vi "CR-SaveImage -CCD3NG.vi"(6 "CCD Name":string(combo), 8 "error in (no error)":errorcluster, 9 "Image in":T1(plugin-control), 10 "布尔":bool=TRUE, 11 "基路径":path) -> (0 "error out":errorcluster)   [LabVIEW 2017]
panel:
  out "连接的字符串":string
  # "D:\\Data\\History Image\\20190228\\CCD3\\Image"
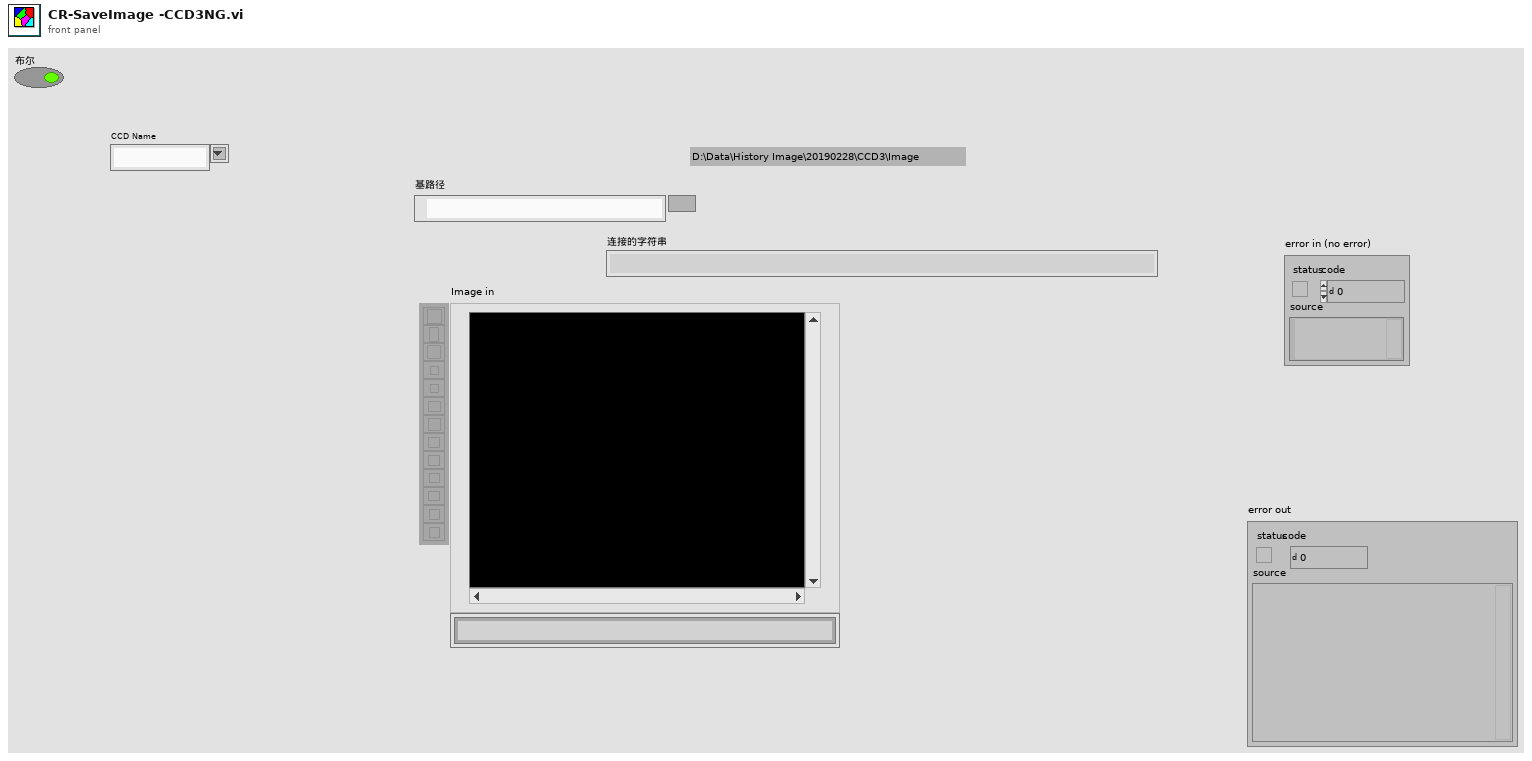
[diagram p1: front panel]
types:
  T1 = typedef "IMAQ Image.ctl" = refnum<image>
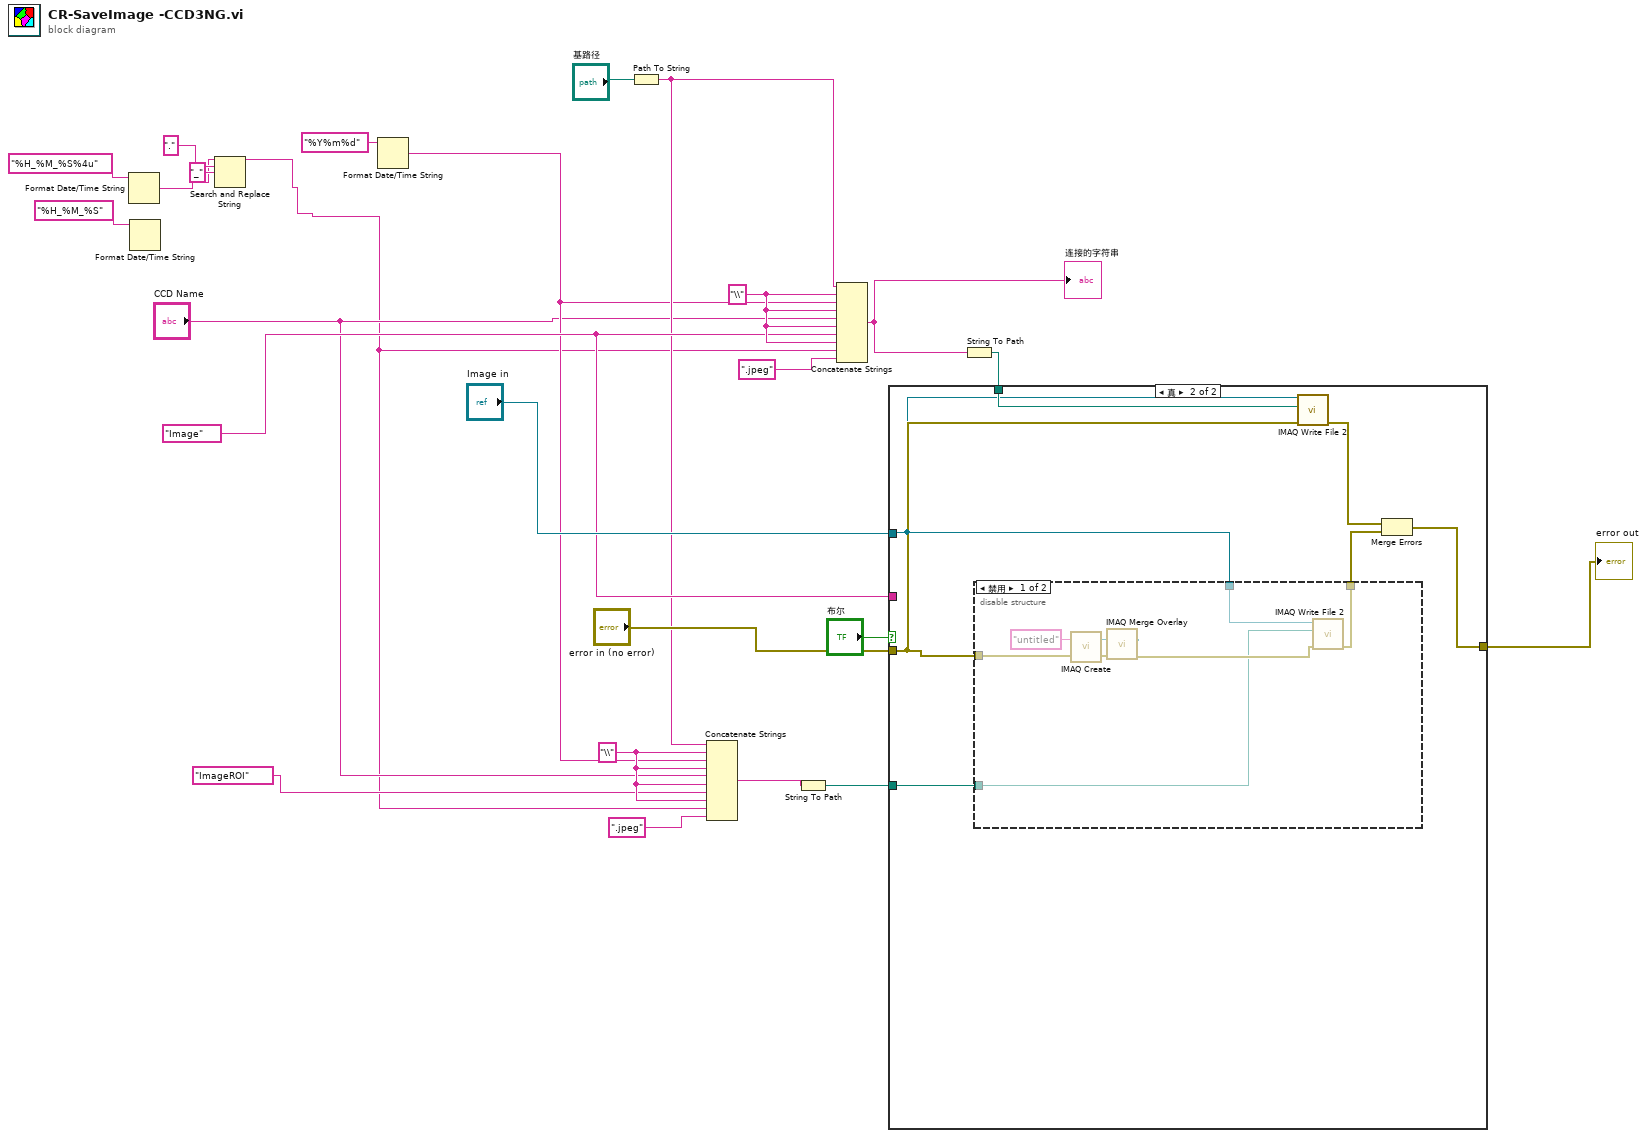
[diagram p0: block diagram]
diagram:
  w16 = "Image" ("类型")
  w14 = "\\" ("字符串")
  w18 = "\\" ("字符串")
  n1 = Format Date/Time String(time format string (%c)="%H_%M_%S%4u" ("时间格式字符串(%c)")) -> (date/time string=w3:string)  [unwired: 2 in]
  n2 = Format Date/Time String(time format string (%c)="%H_%M_%S" ("时间格式字符串(%c)")) -> ()  [unwired: 2 in, 1 out]
  n3 = Search and Replace String(input string=w3, search string="." ("搜索字符串"), replace string="_" ("替换字符串(\"\")")) -> (result string=w1:string)  [unwired: 5 in, 3 out]
  n4 = Format Date/Time String(time format string (%c)="%Y%m%d" ("时间格式字符串(%c)")) -> (date/time string=w11:string)  [unwired: 2 in]
  n5 = Path To String(path="基路径") -> (string=w12:string)
  n6 = Concatenate Strings(w12, w14, w11, w14, "CCD Name", w14, "ImageROI" ("类型"), w14, w1, ".jpeg" ("字符串")) -> (w8:string)
  n7 = String To Path(string=w8) -> (path=w7:path)
  n8 = Concatenate Strings(w12, w18, w11, w18, "CCD Name", w18, w16, w18, w1, ".jpeg" ("字符串")) -> (w24:string)
  "连接的字符串" <- w24
  n9 = String To Path(string=w24) -> (path=w20:path)
  n10 = case shown="真" "布尔" {
    tunnel: "Image in" -> [_ w27]
    tunnel: "error in (no error)" -> [w26 w33]
    tunnel: w20 -> [_ w28]
    tunnel: [w26 w30] -> w17
    tunnel: w16 -> [_ _]
    tunnel: w7 -> [_ w29]
    frame False {
    }
    frame True {
      n11 = disable-structure shown="禁用" {
        disable-tunnel: w33 -> [w41 _]
        disable-tunnel: [w39 _] -> w32
        disable-tunnel: w29 -> [w38 _]
        disable-tunnel: w27 -> [w37 _]
        frame Disabled {
          n12 = call "IMAQ Create"("Image Name"="untitled", "error in (no error)"=w41) -> ("New Image"=w35:T1, "error out"=w34:errorcluster)  [unwired: 3 in]
          n13 = call "IMAQ Merge Overlay"("error in (no error)"=w34, "Image Dst"=w35) -> ("error out"=w40:errorcluster)  [unwired: 8 in, 1 out]
          n14 = call-poly "IMAQ Write File 2"("error in (no error)"=w40, "File Path"=w38, "Image"=w37) -> ("error out"=w39:errorcluster)  [unwired: 7 in, 1 out]
        }
        frame Enabled {
        }
      }
      n15 = call-poly "IMAQ Write File 2"("error in (no error)"=w33, "File Path"=w28, "Image"=w27) -> ("error out"=w31:errorcluster)  [unwired: 7 in, 1 out]
      n16 = Merge Errors(w31, w32) -> (w30:errorcluster)
    }
  }
  "error out" <- w17
